vi "generate_VS.vi"(1 "Analog Out Channels":cluster{"0":bool, "1":bool}={"0"=TRUE, "1"=FALSE}, 2 "Generate config":T1={"maximum value"=5.0, "minimum value"=-5.0, "phase"=180.0, "amplitude"=1.0, "frequency"=10.0, "Wave Type"=0, "offset"=0.0} {"offset" format="%0.2p"; "Wave Type" items=["Sine", "Square", "Triangle", "Sawtooth", "DC Signal"]; "frequency" format="%0.2p"; "amplitude" format="%0.2p"}) -> (0 "signal Generated":waveform(dbl)(graph))   [LabVIEW 2017]
uses:
  <vilib>/DAQmx/write.llb/DAQmx Write (Analog Wfm 1Chan NSamp).vi
  <vilib>/DAQmx/create/channels.llb/DAQmx Create Channel (AO-Voltage-Basic).vi
  <vilib>/DAQmx/configure/timing.llb/DAQmx Timing (Use Waveform).vi
  <vilib>/DAQmx/miscellaneous.llb/DAQmx Fill In Error Info.vi
  <instrlib>/NI USB-6356/NI USB-6356.lvlib
panel:
  out "real frequency(Hz)":dbl
  in  "error in":errorcluster
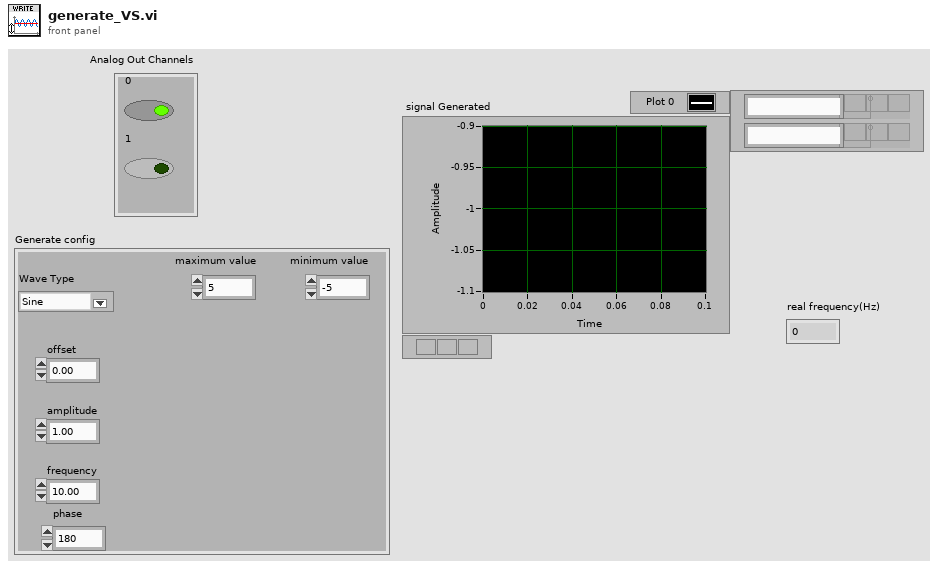
[diagram p1: front panel]
types:
  T1 = cluster{"maximum value":dbl, "minimum value":dbl, "phase":dbl, "amplitude":dbl, "frequency":dbl, "Wave Type":u16, "offset":dbl}
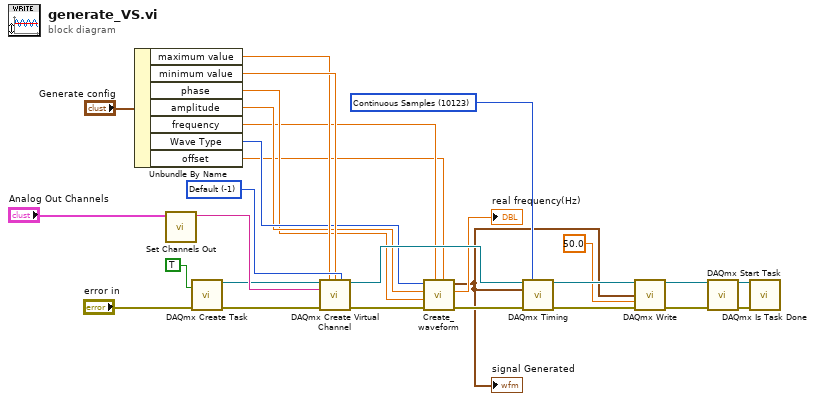
[diagram p0: block diagram]
diagram:
  w22 = 10123 items=["Finite Samples"=10178, "Continuous Samples"=10123, "Hardware Timed Single Point"=12522] ("sample mode")
  w28 = -1 items=["Default"=-1, "RSE"=10083, "Differential"=10106, "Pseudodifferential"=12529] ("output terminal configuration")
  n1 = Unbundle By Name("Generate config") -> ("maximum value"=w6:dbl, "minimum value"=w7:dbl, "phase"=w3:dbl, "amplitude"=w4:dbl, "frequency"=w2:dbl, "Wave Type"=w5:u16, "offset"=w1:dbl)
  n2 = call <instrlib>:"Set Channels Out.vi"("Analog Out Channels"="Analog Out Channels") -> ("String"=w27:string)  [unwired: 10 in]
  n3 = call <vilib>:"DAQmx Create Task.vi"("auto cleanup"=TRUE, "error in"="error in") -> ("task out"=w13:refnum<k21>, "error out"=w12:errorcluster)  [unwired: 12 in]
  n4 = call-poly <vilib>:"DAQmx Create Virtual Channel.vi"("task in"=w13, "maximum value"=w6, "minimum value"=w7, "output terminal configuration"=w28, "physical channels"=w27, "error in"=w12) -> ("task out"=w26:refnum<k21>, "error out"=w25:errorcluster)  [unwired: 8 in]
  n5 = call "Create_waveform.vi"("offset"=w1, "frequency"=w2, "error in"=w25, "phase"=w3, "amplitude"=w4, "Wave Type"=w5) -> ("error out"=w16:errorcluster, "real frequency(Hz)"=→"real frequency(Hz)":dbl, "signal Generated"=w9:waveform(dbl))  [unwired: 3 in]
  "signal Generated" <- w9
  n6 = call-poly <vilib>:"DAQmx Timing.vi"("task/channels in"=w26, "sample mode"=w22, "waveform"=w9, "error in"=w16) -> ("task out"=w23:refnum<k21>, "error out"=w24:errorcluster)  [unwired: 10 in]
  n7 = call-poly <vilib>:"DAQmx Write.vi"("task/channels in"=w23, "data"=w9, "timeout"=50.0, "error in"=w24) -> ("task out"=w20:refnum<k21>, "error out"=w19:errorcluster)  [unwired: 9 in, 1 out]
  n8 = call <vilib>:"DAQmx Start Task.vi"("task/channels in"=w20, "error in"=w19) -> ("task out"=w18:refnum<k21>, "error out"=w17:errorcluster)  [unwired: 12 in]
  n9 = call <vilib>:"DAQmx Is Task Done.vi"("task/channels in"=w18, "error in"=w17) -> ()  [unwired: 11 in, 3 out]
